vi "LOG DI.vi"(0 "tdms file in":refnum<k34>, 3 "error in":errorcluster, 4 "DI_queue":refnum<queue>) -> (7 "tdms file out":refnum<k34>, 10 "error out":errorcluster)   [LabVIEW 2022 SP3]
uses:
  <vilib>/Waveform/DWDTOps.llb/DWDT Digital to Analog.vi
  <vilib>/Waveform/DWDTOps.llb/DWDT Get Waveform Time Array.vi
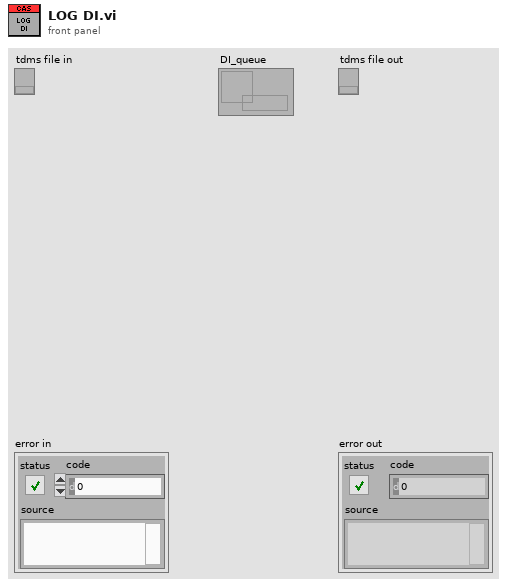
[diagram p1: front panel]
types:
  T1 = cluster{"AO Names":string[], "AI Names":string[], "DI Names":string[], "DO Names":string[], "TC Names":string[], "AO Default":dbl[], "DO Default":bool[], "ACC Names":string[], "SG Names":string[]}
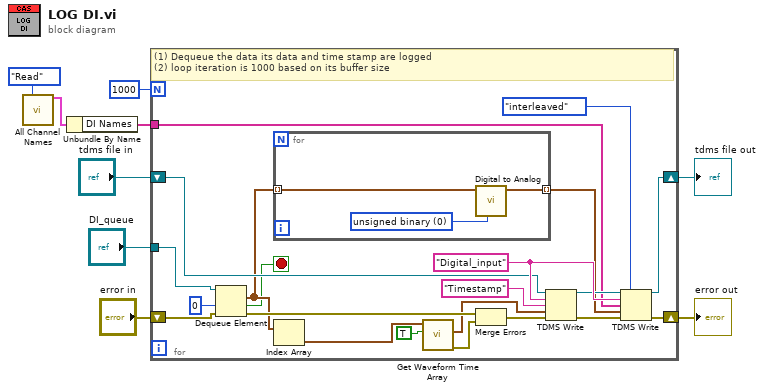
[diagram p0: block diagram]
diagram:
  n1 = call "All Channel Names.vi"("Enum"=enum16{"Read", "Write"}."Read") -> ("Channel names"=w3:T1)  [unwired: 13 in, 1 out]
  n2 = Unbundle By Name(w3) -> ("DI Names"=w2:string[])
  n3 = for {
    N: 1000 -> [_]
    shift-right: [w18] -> w5
    shift-left: "tdms file in" -> [w20]
    shift-right: [w24] -> w4
    shift-left: "error in" -> [w27]
    tunnel: "DI_queue" -> [w11]
    tunnel: w2 -> [w10]
    stop <- w14 stop-if-true
    w23 = "Digital_input" ("group name in (Untitled)")
    # "(1) Dequeue the data its data and time stamp are logged\n(2) loop iteration is 1000 based on its buffer size"
    n4 = Dequeue Element(queue=w11, timeout in ms (-1)=0, error in (no error)=w27) -> (element=w16:digitalwaveform[], timed out?=w14:bool, error out=w29:errorcluster)  [unwired: 1 out]
    n5 = for {
      tunnel: w16 -> [w33] mode=indexing
      tunnel: [w32] -> w15 mode=indexing
      w31 = u16 0 items=["unsigned binary", "offset binary", "2's complement"] ("data format (offset binary)")
      n6 = call-poly <vilib>:"Digital to Analog.vi"("data format (offset binary)"=w31, "digital waveform"=w33) -> ("analog waveform"=w32:waveform(dbl))  [unwired: 6 in, 3 out]
    }
    n7 = Index Array(array=w16) -> (element=w12:digitalwaveform)  [unwired: 1 in]
    n8 = call-poly <vilib>:"Get Waveform Time Array.vi"("match transition array"=TRUE, "waveform in"=w12) -> ("error out"=w28:errorcluster, "X array"=w21:timestamp[])  [unwired: 8 in]
    n9 = Merge Errors(w29, w28) -> (w26:errorcluster)
    n10 = TDMS Write(0:w20, 5:w23, 7:"Timestamp", 9:w21, 11:w26) -> (4:w19:refnum<k34>, 15:w25:errorcluster)  [unwired: 1 in, 2 out]
    n11 = TDMS Write(0:w19, 1:enum16{"decimated", "interleaved"}."interleaved" ("data layout (0:decimated)"), 5:w23, 7:w10, 9:w15, 11:w25) -> (4:w18:refnum<k34>, 15:w24:errorcluster)  [unwired: 2 out]
  }
  "tdms file out" <- w5
  "error out" <- w4
